vi "load configuration from database by ID.vi"(8 "error in":errorcluster, 10 "ID":string, 11 "database in":T1[](array[typedef])) -> (0 "error out":errorcluster, 2 "configuration":refnum<class "TBM configuration.lvclass">, 3 "database out":T1[](array[typedef]))   [LabVIEW 2013, in "PLConfigurationSerializer.lvlib"]
uses:
  PLConfigurationSerializer.lvlib
  configuration database.ctl
  <vilib>/NI/Tag Bus Module Framework/root configuration/TBM configuration.lvclass
  <vilib>/NI/CEF/CEF_TreeControl/NISE_CEF_TreeControl.lvlib
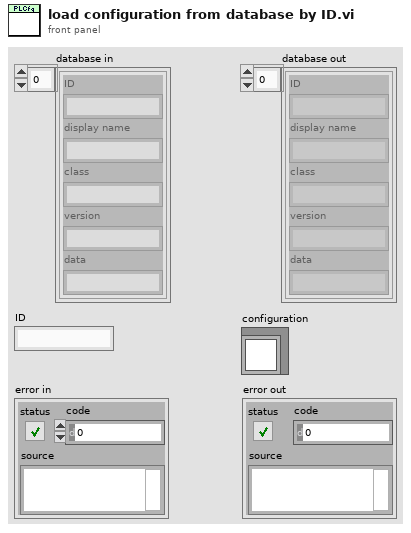
[diagram p1: front panel]
types:
  T1 = typedef "PLConfigurationSerializer.lvlib/configuration database.ctl" = cluster{"ID":string, "display name":string, "class":string, "version":string, "data":string}
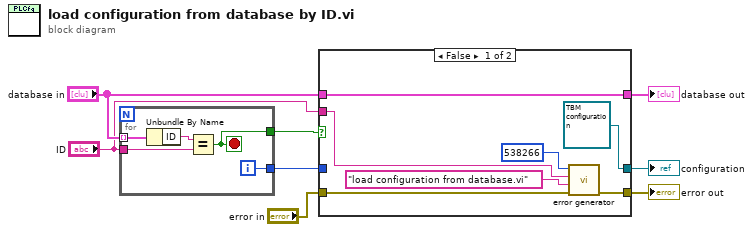
[diagram p0: block diagram]
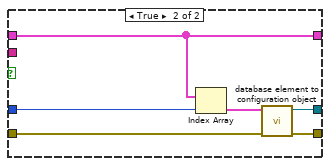
[diagram p2: hidden frame]
diagram:
  n1 = for {
    tunnel: "database in" -> [w11] mode=indexing
    tunnel: "ID" -> [w12]
    tunnel: [w10] -> w3
    tunnel: [w9] -> w2
    i -> [w9]
    stop <- w10 stop-if-true
    n2 = Unbundle By Name(w11) -> ("ID"=w13:string)
    n3 = Equal?(x=w13, y=w12) -> (x = y?=w10:bool)
  }
  n4 = case shown="False" w3 {
    tunnel: [refnum<class "TBM configuration.lvclass"> refnum ("configuration in") w26] -> w8
    tunnel: "error in" -> [w18 w25]
    tunnel: [w17 w24] -> w6
    tunnel: [w19 w23] -> w5
    tunnel: "database in" -> [w19 w23]
    tunnel: w2 -> [_ w22]
    tunnel: "ID" -> [w16 _]
    frame False {
      n5 = call <vilib>:"error generator.vi"("error in"=w18, "source"="load configuration from database.vi", "append error message"=w16, "error code (0)"=538266) -> ("error out"=w17:errorcluster)  [unwired: 5 in]
    }
    frame True {
      n6 = Index Array(array=w23, index=w22) -> (element=w21:T1)
      n7 = call "database element to configuration object.vi"("error in"=w25, "database"=w21) -> ("error out"=w24:errorcluster, "configuration in"=w26:refnum<class "TBM configuration.lvclass">)  [unwired: 8 in]
    }
  }
  "database out" <- w5
  "configuration" <- w8
  "error out" <- w6
